vi "pco.camera_Live_Example_IMAQ - Copy.vi"() -> ()   [LabVIEW 2020]
doc: "A short program to demonstrate the fundamentals of control and image acquision with the pco.camera series. The program records a sequence of images, with \"live\" updating, until the \"StopRecording\" button is pressed. Use ctrl-H for more help on the individual controls and indicators.\n\nCopyright 2004, 2010 The Cooke Corporation."
uses:
  Camera.lvclass
  TimingControl.lvlib
panel:
  in  "Trigger":bool
  in  "data_format":T1(ring)=enum."Mono16"
  out "Image":T2(plugin-control)
  out "rawImage":u16[][](array[numeric])
  in  "Image Index":u32 max=9
  out "Recorded Images":u32
  in  "TriggerMode":T3(ring)
  in  "Quit":bool
  out "Error":errorcluster {"code" format="%x"}
  in  "Stop Record":bool
  out "Recording On":bool
  in  "roiY1":u64=2 min=1 max=1040 step=1
  in  "roiX1":u64=2 min=1 max=1392 step=1
  in  "roiY0":u64=1 min=1 max=1039 step=1
  in  "roiX0":u64=1 min=1 max=1391 step=1
  out "Image Height":u64
  out "Image Width":u64
  in  "dwImgCount":u32=10 caption="Required Number of Images" max=2397
  in  "Exposure Time [s]":dbl=0.010000000000000002 min=1e-06 max=60.0 step=0.001
  # "This example demonstrates the image acquisition with one camera in ring buffer mode together with a live display of the latest images during record. After record is stopped, the images can be addressed by index.\nNote that this example will not be fail save, i.e. doesnt react on errors, just handles them forward to the end\n\nUsage:\nSelect your required image count, data format and the camera setup before you start the program.\nOnce started, the camera class will be initialized and images will be recorded and displayed automatically\nYou can stop the images by pressing stop record.\nAfter stopped, the image at the selected index will be read out\nTo finish the program click on quit application, this will force an exit of the camera class\nYou can change your required ROI after and also during the record."
  # "pco.labview"
  # "Camera Setup"
  # "Recording Control"
  # "Parameters for image readout"
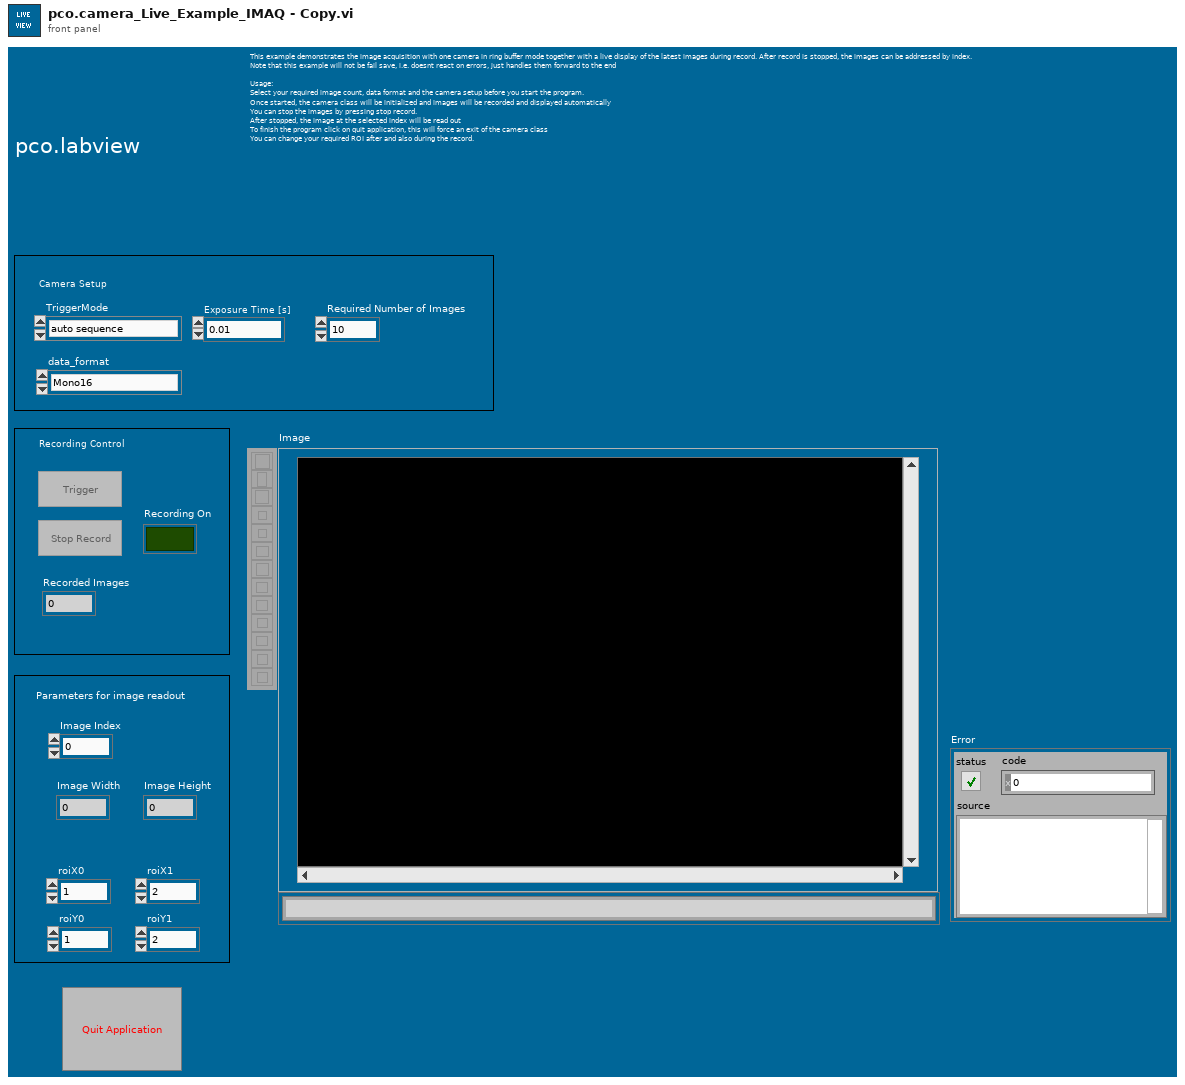
[diagram p1: front panel]
types:
  T1 = enum16{"Undefined", "Mono8", "Mono16", "BGRA8", "RGBA8", "BGRA16", "RGBA16", "CompressedMono8"}
  T2 = typedef "IMAQ Image.ctl" = refnum<image>
  T3 = enum16{"auto sequence", "software trigger", "external exposure start", "external exposure control"}
  T4 = enum16{"sequence", "sequence non blocking", "ring buffer", "fifo", "sequence_dpcore", "sequence_non_blocking_dpcore", "ring_buffer_dpcore", "fifo_dpcore", "tif", "multitif", "pcoraw", "b16", "dicom", "multidicom"}
  T5 = enum8{"Enabled", "Disabled", "Disabled and Grayed Out"}
  T6 = cluster{"serial":u32, "type":u16, "sub_type":u16, "interface_type":u16, "bit_resolution":u16, "min_exposure_time_s":dbl, "max_exposure_time_s":dbl, "min_exposure_step_s":dbl, "min_delay_time_s":dbl, "max_delay_time_s":dbl, "min_delay_step_s":dbl, "min_width":u64, "min_height":u64, "max_width":u64, "max_height":u64, "roi_step_horz":u64, "roi_step_vert":u64, "roi_symmetric_horz":bool, "roi_symmetric_vert":bool, "has_timestamp_mode":bool, "has_timestamp_mode_ascii_only":bool, "pixelrate_vec":u32[], "has_acquire_mode":bool, "has_ext_acquire_mode":bool, "has_metadata_mode":bool, "has_ram":bool, "binning_horz_vec":u16[], "binning_vert_vec":u16[]}
  T7 = typedef "Image Type" = u32
  T8 = typedef "Camera.lvclass/binning.ctl" = cluster{"vert":u16, "horz":u16}
  T9 = cluster{"exposure_time_s":dbl, "delay_time_s":dbl, "roi":cluster{"x0":u64, "y0":u64, "x1":u64, "y1":u64}, "timestamp_mode":u16, "pixelrate":u32, "trigger_mode":u16, "acquire_mode":u16, "metadata_mode":u16, "noisefilter_mode":u16, "binning":T8}
  T10 = cluster{"Plane 4 (alpha)":u16, "Plane 1 (Red)":u16, "Plane 2 (Green)":u16, "Plane 3 (Blue)":u16}[][]
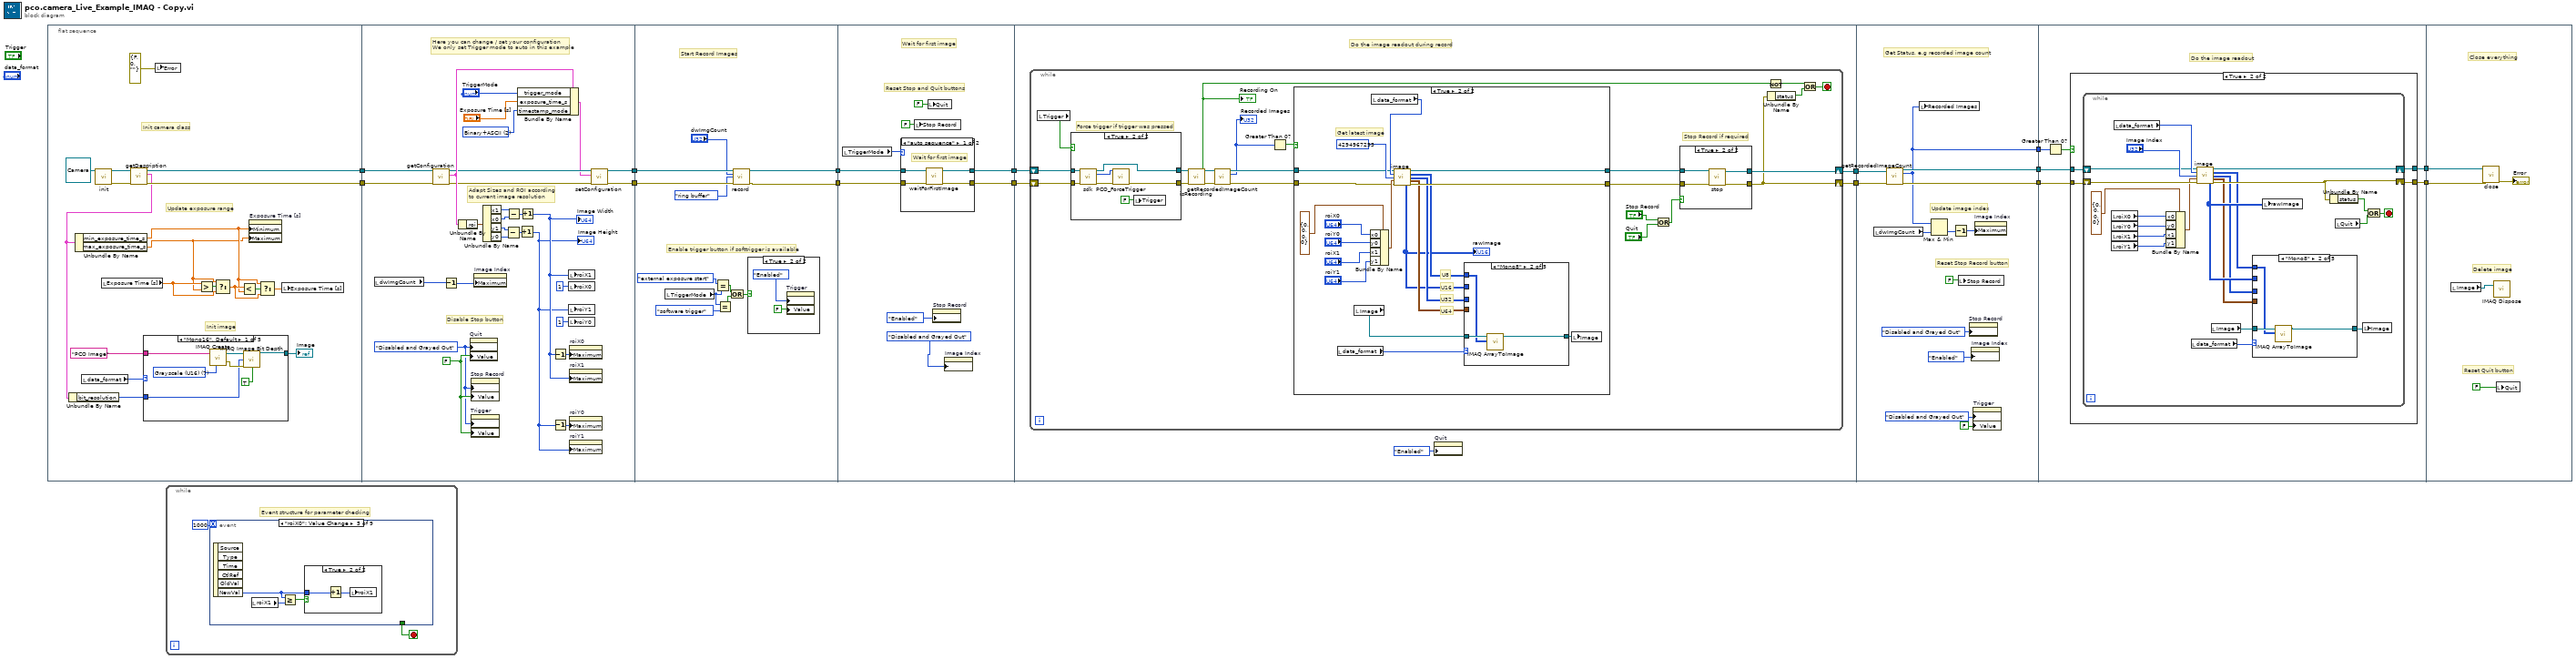
[diagram p0: block diagram]
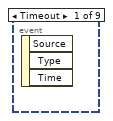
[diagram p2: hidden frame]
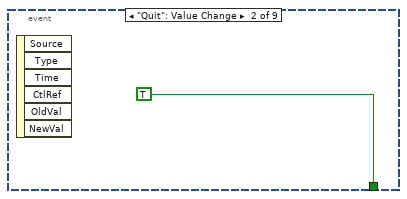
[diagram p3: hidden frame]
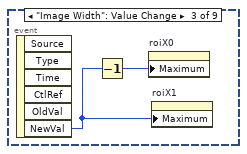
[diagram p4: hidden frame]
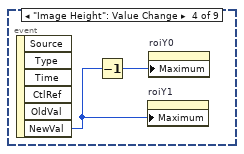
[diagram p5: hidden frame]
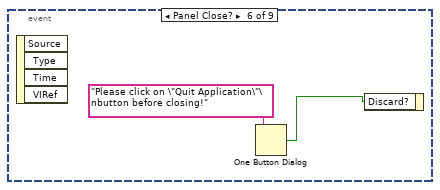
[diagram p7: hidden frame]
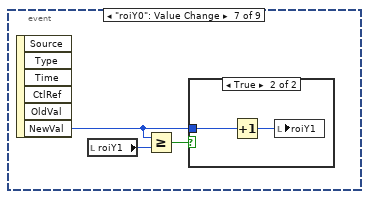
[diagram p8: hidden frame]
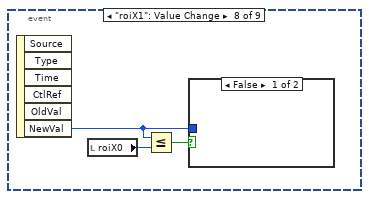
[diagram p10: hidden frame]
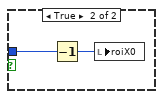
[diagram p11: hidden frame]
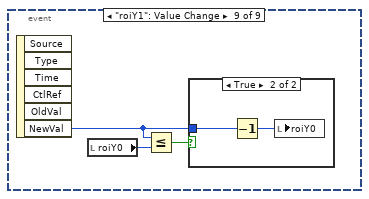
[diagram p12: hidden frame]
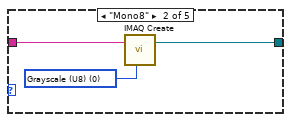
[diagram p14: hidden frame]
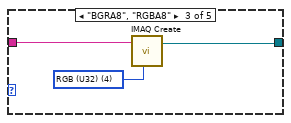
[diagram p15: hidden frame]
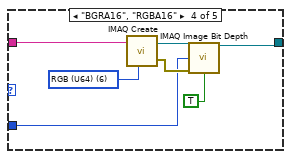
[diagram p16: hidden frame]
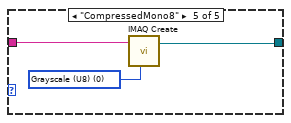
[diagram p17: hidden frame]
diagram:
  n1 = flat-sequence {
    tunnel: [w22] -> w7
    tunnel: [w21] -> w6
    tunnel: [w61] -> w15
    tunnel: [w65] -> w14
    tunnel: w7 -> [w60]
    tunnel: w6 -> [w59]
    tunnel: [w85] -> w9
    tunnel: [w86] -> w8
    tunnel: w14 -> [w96]
    tunnel: w15 -> [w95]
    tunnel: w9 -> [w103]
    tunnel: w8 -> [w104]
    tunnel: [w102] -> w13
    tunnel: [w100] -> w2
    tunnel: w13 -> [w118]
    tunnel: [w116] -> w12
    tunnel: [w115] -> w5
    tunnel: w2 -> [w114]
    tunnel: w12 -> [w201]
    tunnel: [w199] -> w11
    tunnel: w5 -> [w194]
    tunnel: [w193] -> w4
    tunnel: [w192] -> w1
    tunnel: w11 -> [w210]
    tunnel: [w209] -> w10
    tunnel: w4 -> [w208]
    tunnel: [w207] -> w3
    tunnel: w1 -> [w205]
    tunnel: w10 -> [w257]
    tunnel: w3 -> [w255]
    frame #0 {
      # "Init image"
      # "Init camera class"
      # "Update exposure range"
      n2 = local read "data_format"() -> (w18:T1)
      n3 = call-dynamic "init.vi"("Camera in"=refnum<class "Camera.lvclass"> refnum) -> ("Camera out"=w23:refnum<class "Camera.lvclass">, "error out"=w24:errorcluster)  [unwired: 8 in]
      n4 = local read "Exposure Time [s]"() -> (w32:dbl)
      n5 = call-dynamic "getDescription.vi"("error in (no error)"=w24, "Camera in"=w23) -> ("error out"=w21:errorcluster, "description"=w17:T6, "Camera out"=w22:refnum<class "Camera.lvclass">)  [unwired: 7 in]
      n6 = Unbundle By Name(w17) -> ("bit_resolution"=w16:u16)
      n7 = Unbundle By Name(w17) -> ("min_exposure_time_s"=w20:dbl, "max_exposure_time_s"=w19:dbl)
      n8 = case shown="\"Mono16\", Default" w18 {
        tunnel: "PCO Image" ("Image Name") -> [w39 w43 w45 w52 w55]
        tunnel: [w35 w41 w44 w49 w54] -> w25
        tunnel: w16 -> [w34 _ _ w47 _]
        frame "Mono16", Default {
          w40 = T7 7 items=["Grayscale (U8)", "Grayscale (I16)", "Grayscale (SGL)", "Complex (CSG)", "RGB (U32)", "HSL (U32)", "RGB (U64)", "Grayscale (U16)"] ("Image Type")
          n9 = call "IMAQ Create"("Image Name"=w39, "Image Type"=w40) -> ("New Image"=w37:T2, "error out"=w36:errorcluster)  [unwired: 3 in]
          n10 = call "IMAQ Image Bit Depth"("Image"=w37, "Bit Depth (0)"=w34, "error in (no error)"=w36, "Get/Set Bit Depth? (Set)"=TRUE) -> ("Image Out"=w35:T2)  [unwired: 9 in, 2 out]
        }
        frame "Mono8" {
          w42 = T7 0 items=["Grayscale (U8)", "Grayscale (I16)", "Grayscale (SGL)", "Complex (CSG)", "RGB (U32)", "HSL (U32)", "RGB (U64)", "Grayscale (U16)"] ("Image Type")
          n11 = call "IMAQ Create"("Image Name"=w43, "Image Type"=w42) -> ("New Image"=w41:T2)  [unwired: 3 in, 1 out]
        }
        frame "BGRA8", "RGBA8" {
          w46 = T7 4 items=["Grayscale (U8)", "Grayscale (I16)", "Grayscale (SGL)", "Complex (CSG)", "RGB (U32)", "HSL (U32)", "RGB (U64)", "Grayscale (U16)"] ("Image Type")
          n12 = call "IMAQ Create"("Image Name"=w45, "Image Type"=w46) -> ("New Image"=w44:T2)  [unwired: 3 in, 1 out]
        }
        frame "BGRA16", "RGBA16" {
          w53 = T7 6 items=["Grayscale (U8)", "Grayscale (I16)", "Grayscale (SGL)", "Complex (CSG)", "RGB (U32)", "HSL (U32)", "RGB (U64)", "Grayscale (U16)"] ("Image Type")
          n13 = call "IMAQ Create"("Image Name"=w52, "Image Type"=w53) -> ("New Image"=w50:T2, "error out"=w48:errorcluster)  [unwired: 3 in]
          n14 = call "IMAQ Image Bit Depth"("Image"=w50, "Bit Depth (0)"=w47, "error in (no error)"=w48, "Get/Set Bit Depth? (Set)"=TRUE) -> ("Image Out"=w49:T2)  [unwired: 9 in, 2 out]
        }
        frame "CompressedMono8" {
          w56 = T7 0 items=["Grayscale (U8)", "Grayscale (I16)", "Grayscale (SGL)", "Complex (CSG)", "RGB (U32)", "HSL (U32)", "RGB (U64)", "Grayscale (U16)"] ("Image Type")
          n15 = call "IMAQ Create"("Image Name"=w55, "Image Type"=w56) -> ("New Image"=w54:T2)  [unwired: 3 in, 1 out]
        }
      }
      "Image" <- w25
      n16 = local write "Error"(errorcluster {"status"=FALSE, "code"=0, "source"=""} ("error IO")) -> ()
      n17 = Greater?(x=w32, y=w19) -> (0:w33:bool)
      n18 = Select(t=w19, s=w33, f=w32) -> (s? t:f=w30:dbl)
      n19 = Less?(x=w30, y=w20) -> (x < y?=w31:bool)
      n20 = property on="Exposure Time [s]" class="DigNum (strict)"("Minimum"=w20, "Maximum"=w19) -> ()  [unwired: 2 in, 2 out]
      n21 = Select(t=w20, s=w31, f=w30) -> (s? t:f=w29:dbl)
      n22 = local write "Exposure Time [s]"(w29) -> ()
    }
    frame #1 {
      w71 = u16 2 items=["OFF", "Binary", "Binary+ASCII", "ASCII"] ("wTimeStampMode")
      w58 = FALSE ("Stop")
      w57 = T5."Disabled and Grayed Out" ("Disabled")
      # "Disable Stop button"
      # "Adapt Sizes and ROI according\nto current image resolution"
      # "Here you can change / set your configuration\nWe only set Trigger mode to auto in this example"
      n23 = local read "dwImgCount"() -> (w72:u32)
      n24 = call-dynamic "getConfiguration.vi"("error in (no error)"=w59, "Camera in"=w60) -> ("error out"=w66:errorcluster, "configuration"=w77:T9, "Camera out"=w68:refnum<class "Camera.lvclass">)  [unwired: 7 in]
      n25 = Decrement(x=w72) -> (x-1=w62:u32)
      n26 = Unbundle By Name(w77) -> ("roi"=w78:cluster{"x0":u64, "y0":u64, "x1":u64, "y1":u64})
      n27 = property on="Quit" class="Bool (strict)"("DisabledEnum"=w57, "Value"=w58) -> ()  [unwired: 2 in, 2 out]
      n28 = property on="Stop Record" class="Bool (strict)"("DisabledEnum"=w57, "Value"=w58) -> ()  [unwired: 2 in, 2 out]
      n29 = property on="Trigger" class="Bool (strict)"("DisabledEnum"=w57, "Value"=w58) -> ()  [unwired: 2 in, 2 out]
      n30 = property on="Image Index" class="DigNum (strict)"("Maximum"=w62) -> ()  [unwired: 2 in, 2 out]
      n31 = Unbundle By Name(w78) -> ("x1"=w80:u64, "x0"=w79:u64, "y1"=w82:u64, "y0"=w81:u64)
      n32 = Subtract(x=w82, y=w81) -> (x-y=w84:u64)
      n33 = Subtract(x=w80, y=w79) -> (x-y=w83:u64)
      n34 = Bundle By Name(cluster=w77, "trigger_mode"="TriggerMode", "exposure_time_s"="Exposure Time [s]", "timestamp_mode"=w71) -> (w67:T9)
      n35 = Increment(x=w84) -> (x+1=w63:u64)
      "Image Height" <- w63
      n36 = Increment(x=w83) -> (x+1=w64:u64)
      "Image Width" <- w64
      n37 = Decrement(x=w64) -> (x-1=w75:u64)
      n38 = Decrement(x=w63) -> (x-1=w76:u64)
      n39 = local write "roiX1"(w64) -> ()
      n40 = local write "roiX0"(u64 1 ("roiY0")) -> ()
      n41 = local write "roiY1"(w63) -> ()
      n42 = local write "roiY0"(u64 1 ("roiY0")) -> ()
      n43 = property on="roiX0" class="DigNum (strict)"("Maximum"=w75) -> ()  [unwired: 2 in, 2 out]
      n44 = property on="roiX1" class="DigNum (strict)"("Maximum"=w64) -> ()  [unwired: 2 in, 2 out]
      n45 = property on="roiY0" class="DigNum (strict)"("Maximum"=w76) -> ()  [unwired: 2 in, 2 out]
      n46 = property on="roiY1" class="DigNum (strict)"("Maximum"=w63) -> ()  [unwired: 2 in, 2 out]
      n47 = call-dynamic "setConfiguration.vi"("error in (no error)"=w66, "configuration"=w67, "Camera in"=w68) -> ("error out"=w65:errorcluster, "Camera out"=w61:refnum<class "Camera.lvclass">)  [unwired: 7 in]
    }
    frame #2 {
      # "Enable trigger button if softtrigger is available"
      # "Start Record Images"
      n48 = local read "TriggerMode"() -> (w92:T3)
      n49 = Equal?(x=T3."external exposure start" ("TriggerMode"), y=w92) -> (x = y?=w89:bool)
      n50 = Equal?(x=w92, y=T3."software trigger" ("TriggerMode")) -> (x = y?=w88:bool)
      n51 = Or(x=w89, y=w88) -> (x .or. y?=w90:bool)
      n52 = call-dynamic "record.vi"("Camera in"=w95, "num_images"="dwImgCount", "record_mode"=T4."ring buffer", "error in (no error)"=w96) -> ("Camera out"=w86:refnum<class "Camera.lvclass">, "error out"=w85:errorcluster)  [unwired: 10 in]
      n53 = case shown="True" w90 {
        frame False {
        }
        frame True {
          n54 = property on="Trigger" class="Bool (strict)"("DisabledEnum"=T5."Enabled" ("Disabled"), "Value"=FALSE ("Trigger")) -> ()  [unwired: 2 in, 2 out]
        }
      }
    }
    frame #3 {
      # "Wait for first image"
      # "Reset Stop and Quit buttons"
      n55 = local read "TriggerMode"() -> (w99:T3)
      n56 = case shown="\"auto sequence\"" w99 {
        tunnel: w104 -> [w111 w113]
        tunnel: w103 -> [w110 w112]
        tunnel: [w109 w112] -> w102
        tunnel: [w108 w113] -> w100
        frame "auto sequence" {
          # "Wait for first image"
          n57 = call-dynamic "waitForFirstImage.vi"("error in (no error)"=w110, "Camera in"=w111) -> ("error out"=w109:errorcluster, "Camera out"=w108:refnum<class "Camera.lvclass">)  [unwired: 8 in]
        }
        frame Default {
        }
      }
      n58 = local write "Stop Record"(FALSE ("Stop Record")) -> ()
      n59 = local write "Quit"(FALSE ("Stop")) -> ()
      n60 = property on="Stop Record" class="Bool (strict)"("DisabledEnum"=T5."Enabled" ("Disabled")) -> ()  [unwired: 2 in, 2 out]
      n61 = property on="Image Index" class="DigNum (strict)"("DisabledEnum"=T5."Disabled and Grayed Out" ("Disabled")) -> ()  [unwired: 2 in, 2 out]
    }
    frame #4 {
      # "Do the image readout during record"
      n62 = while {
        shift-right: [w121] -> w116
        shift-left: w118 -> [w125]
        shift-right: [w122] -> w115
        shift-left: w114 -> [w126]
        stop <- w137 stop-if-true
        # "Force trigger if trigger was pressed"
        # "Stop Record if required"
        n63 = local read "Trigger"() -> (w127:bool)
        n64 = case shown="True" w127 {
          tunnel: w126 -> [w178 w183]
          tunnel: w125 -> [w177 w182]
          tunnel: [w178 w181] -> w124
          tunnel: [w177 w180] -> w123
          frame False {
          }
          frame True {
            n65 = call-dynamic "sdk.vi"("Camera in"=w183, "error in (no error)"=w182) -> ("Camera out"=w181:refnum<class "Camera.lvclass">, "sdk"=w184:u64, "error out"=w185:errorcluster)  [unwired: 11 in]
            n66 = call "PCO_ForceTrigger.vi"("error in (no error)"=w185, "ph"=w184) -> ("error out"=w180:errorcluster)  [unwired: 6 in, 3 out]
            n67 = local write "Trigger"(FALSE ("Trigger")) -> ()
          }
        }
        n68 = call-dynamic "isRecording.vi"("Camera in"=w124, "error in (no error)"=w123) -> ("Camera out"=w132:refnum<class "Camera.lvclass">, "recording"=w135:bool, "error out"=w131:errorcluster)  [unwired: 11 in]
        "Recording On" <- w135
        n69 = call-dynamic "getRecordedImageCount.vi"("Camera in"=w132, "error in (no error)"=w131) -> ("Camera out"=w129:refnum<class "Camera.lvclass">, "recorded_image_count"=w119:u32, "error out"=w130:errorcluster)  [unwired: 11 in]
        "Recorded Images" <- w119
        n70 = Greater Than 0?(x=w119) -> (x > 0?=w120:bool)
        n71 = case shown="True" w120 {
          tunnel: [w141 w156] -> w133
          tunnel: w130 -> [w141 w153]
          tunnel: w129 -> [w142 w144]
          tunnel: [w142 w143] -> w128
          frame False {
          }
          frame True {
            # "U64"
            # "U32"
            # "U8"
            # "U16"
            # "Get latest image"
            n72 = local read "data_format"() -> (w145:T1)
            n73 = local read "Image"() -> (w150:T2)
            n74 = Bundle By Name(cluster=cluster{"x0":u64, "y0":u64, "x1":u64, "y1":u64} {"x0"=0, "y0"=0, "x1"=0, "y1"=0} ("roi"), "x0"="roiX0", "y0"="roiY0", "x1"="roiX1", "y1"="roiY1") -> (w157:cluster{"x0":u64, "y0":u64, "x1":u64, "y1":u64})
            n75 = local read "data_format"() -> (w152:T1)
            n76 = call-dynamic "image.vi"("Camera in"=w144, "data_format"=w152, "image_index"=u32 4294967295 ("dwImgIdx"), "roi"=w157, "error in (no error)"=w153) -> ("Camera out"=w143:refnum<class "Camera.lvclass">, "image (U8)"=w147:u8[][], "image (U32)"=w148:u32[][], "image (U64)"=w149:T10, "raw_image (U16)"=w146:u16[][], "error out"=w156:errorcluster)  [unwired: 3 in, 2 out]
            "rawImage" <- w146
            n77 = case shown="\"Mono8\"" w145 {
              tunnel: w150 -> [w164 w167 w170 w173 w176]
              tunnel: [w162 w165 w169 w171 w175] -> w151
              tunnel: w149 -> [_ _ _ w172 _]
              tunnel: w148 -> [_ _ w168 _ _]
              tunnel: w147 -> [_ w166 _ _ w174]
              tunnel: w146 -> [w163 _ _ _ _]
              frame "Mono16", Default {
                n78 = call "IMAQ ArrayToImage"("Image Pixels (U16)"=w163, "Image"=w164) -> ("Image Out"=w162:T2)  [unwired: 8 in, 1 out]
              }
              frame "Mono8" {
                n79 = call "IMAQ ArrayToImage"("Image Pixels (U8)"=w166, "Image"=w167) -> ("Image Out"=w165:T2)  [unwired: 8 in, 1 out]
              }
              frame "BGRA8", "RGBA8" {
                n80 = call "IMAQ ArrayToColorImage"("Image Pixels (U32)"=w168, "Image"=w170) -> ("Image Out"=w169:T2)  [unwired: 3 in, 1 out]
              }
              frame "BGRA16", "RGBA16" {
                n81 = call "IMAQ ArrayToColorImage"("Image"=w173, "Image Pixels (U64)"=w172) -> ("Image Out"=w171:T2)  [unwired: 3 in, 1 out]
              }
              frame "CompressedMono8" {
                n82 = call "IMAQ ArrayToImage"("Image Pixels (U8)"=w174, "Image"=w176) -> ("Image Out"=w175:T2)  [unwired: 8 in, 1 out]
              }
            }
            n83 = local write "Image"(w151) -> ()
          }
        }
        n84 = Or(x="Stop Record", y="Quit") -> (x .or. y?=w138:bool)
        n85 = case shown="True" w138 {
          tunnel: w133 -> [w187 w188]
          tunnel: [w186 w190] -> w122
          tunnel: [w187 w191] -> w121
          tunnel: w128 -> [w186 w189]
          frame False {
          }
          frame True {
            n86 = call-dynamic "stop.vi"("error in (no error)"=w188, "Camera in"=w189) -> ("error out"=w191:errorcluster, "Camera out"=w190:refnum<class "Camera.lvclass">)  [unwired: 8 in]
          }
        }
        n87 = Unbundle By Name(w121) -> ("status"=w136:bool)
        n88 = Not(x=w135) -> (.not. x?=w134:bool)
        n89 = Or(x=w134, y=w136) -> (x .or. y?=w137:bool)
      }
      n90 = property on="Quit" class="Bool (strict)"("DisabledEnum"=T5."Enabled" ("Disabled")) -> ()  [unwired: 2 in, 2 out]
    }
    frame #5 {
      # "Update image index"
      # "Reset Stop Record button"
      # "Get Status, e.g recorded image count"
      n91 = local read "dwImgCount"() -> (w200:u32)
      n92 = call-dynamic "getRecordedImageCount.vi"("Camera in"=w194, "error in (no error)"=w201) -> ("Camera out"=w193:refnum<class "Camera.lvclass">, "recorded_image_count"=w192:u32, "error out"=w199:errorcluster)  [unwired: 11 in]
      n93 = local write "Recorded Images"(w192) -> ()
      n94 = Max & Min(x=w192, y=w200) -> (min(x,y)=w202:u32)  [unwired: 1 out]
      n95 = Decrement(x=w202) -> (x-1=w197:u32)
      n96 = local write "Stop Record"(FALSE ("Stop Record")) -> ()
      n97 = property on="Stop Record" class="Bool (strict)"("DisabledEnum"=T5."Disabled and Grayed Out" ("Disabled")) -> ()  [unwired: 2 in, 2 out]
      n98 = property on="Image Index" class="DigNum (strict)"("DisabledEnum"=T5."Enabled" ("Disabled")) -> ()  [unwired: 2 in, 2 out]
      n99 = property on="Trigger" class="Bool (strict)"("DisabledEnum"=T5."Disabled and Grayed Out" ("Disabled"), "Value"=FALSE ("Trigger")) -> ()  [unwired: 2 in, 2 out]
      n100 = property on="Image Index" class="DigNum (strict)"("Maximum"=w197) -> ()  [unwired: 2 in, 2 out]
    }
    frame #6 {
      # "Do the image readout"
      n101 = Greater Than 0?(x=w205) -> (x > 0?=w206:bool)
      n102 = case shown="True" w206 {
        tunnel: w210 -> [w211 w216]
        tunnel: [w211 w215] -> w209
        tunnel: w208 -> [w212 w214]
        tunnel: [w212 w213] -> w207
        frame False {
        }
        frame True {
          n103 = while {
            shift-right: [w230] -> w215
            shift-left: w216 -> [w238]
            shift-right: [w217] -> w213
            shift-left: w214 -> [w218]
            stop <- w232 stop-if-true
            n104 = local read "roiX0"() -> (w228:u64)
            n105 = local read "roiY0"() -> (w229:u64)
            n106 = local read "roiX1"() -> (w236:u64)
            n107 = local read "roiY1"() -> (w235:u64)
            n108 = local read "data_format"() -> (w226:T1)
            n109 = Bundle By Name(cluster=cluster{"x0":u64, "y0":u64, "x1":u64, "y1":u64} {"x0"=0, "y0"=0, "x1"=0, "y1"=0} ("roi"), "x0"=w228, "y0"=w229, "x1"=w236, "y1"=w235) -> (w237:cluster{"x0":u64, "y0":u64, "x1":u64, "y1":u64})
            n110 = local read "data_format"() -> (w219:T1)
            n111 = call-dynamic "image.vi"("Camera in"=w218, "data_format"=w226, "image_index"="Image Index", "roi"=w237, "error in (no error)"=w238) -> ("Camera out"=w217:refnum<class "Camera.lvclass">, "image (U8)"=w222:u8[][], "image (U32)"=w221:u32[][], "image (U64)"=w220:T10, "raw_image (U16)"=w223:u16[][], "error out"=w230:errorcluster)  [unwired: 3 in, 2 out]
            n112 = local read "Image"() -> (w224:T2)
            n113 = case shown="\"Mono8\"" w219 {
              tunnel: w224 -> [w241 w244 w247 w250 w253]
              tunnel: [w239 w242 w246 w248 w252] -> w225
              tunnel: w220 -> [_ _ _ w249 _]
              tunnel: w221 -> [_ _ w245 _ _]
              tunnel: w222 -> [_ w243 _ _ w251]
              tunnel: w223 -> [w240 _ _ _ _]
              frame "Mono16", Default {
                n114 = call "IMAQ ArrayToImage"("Image Pixels (U16)"=w240, "Image"=w241) -> ("Image Out"=w239:T2)  [unwired: 8 in, 1 out]
              }
              frame "Mono8" {
                n115 = call "IMAQ ArrayToImage"("Image Pixels (U8)"=w243, "Image"=w244) -> ("Image Out"=w242:T2)  [unwired: 8 in, 1 out]
              }
              frame "BGRA8", "RGBA8" {
                n116 = call "IMAQ ArrayToColorImage"("Image Pixels (U32)"=w245, "Image"=w247) -> ("Image Out"=w246:T2)  [unwired: 3 in, 1 out]
              }
              frame "BGRA16", "RGBA16" {
                n117 = call "IMAQ ArrayToColorImage"("Image"=w250, "Image Pixels (U64)"=w249) -> ("Image Out"=w248:T2)  [unwired: 3 in, 1 out]
              }
              frame "CompressedMono8" {
                n118 = call "IMAQ ArrayToImage"("Image Pixels (U8)"=w251, "Image"=w253) -> ("Image Out"=w252:T2)  [unwired: 8 in, 1 out]
              }
            }
            n119 = local write "rawImage"(w223) -> ()
            n120 = Unbundle By Name(w230) -> ("status"=w233:bool)
            n121 = local read "Quit"() -> (w234:bool)
            n122 = local write "Image"(w225) -> ()
            n123 = Or(x=w233, y=w234) -> (x .or. y?=w232:bool)
          }
        }
      }
    }
    frame #7 {
      # "Delete image"
      # "Close everything"
      # "Reset Quit button"
      n124 = local read "Image"() -> (w254:T2)
      n125 = call-dynamic "close.vi"("error in (no error)"=w257, "Camera in"=w255) -> ("error out"=→"Error":errorcluster)  [unwired: 9 in]
      n126 = call "IMAQ Dispose"("Image"=w254) -> ()  [unwired: 5 in, 1 out]
      n127 = local write "Quit"(FALSE ("Stop Record")) -> ()
    }
  }
  n128 = while {
    stop <- w259 stop-if-true
    # "Event structure for parameter checking"
    n129 = event shown="[4] \"roiX0\": Value Change" {
      selector: _ -> [_ _ _ _ _ _ _ _ _]
      dyn-events: _ -> [_ _ _ _ _ _ _ _ _]
      timeout: 1000 -> [_ _ _ _ _ _ _ _ _]
      tunnel: [_ TRUE _ _ _ _ _ _ _] -> w259
      event Timeout {
        n130 = event-data() -> ()  [unwired: 1 in, 3 out]
      }
      event "Quit": Value Change {
        n131 = event-data() -> ()  [unwired: 1 in, 6 out]
      }
      event "Image Width": Value Change {
        n132 = event-data() -> ("NewVal"=w262:u64)  [unwired: 1 in, 5 out]
        n133 = Decrement(x=w262) -> (x-1=w263:u64)
        n134 = property on="roiX0" class="DigNum (strict)"("Maximum"=w263) -> ()  [unwired: 2 in, 2 out]
        n135 = property on="roiX1" class="DigNum (strict)"("Maximum"=w262) -> ()  [unwired: 2 in, 2 out]
      }
      event "Image Height": Value Change {
        n136 = event-data() -> ("NewVal"=w264:u64)  [unwired: 1 in, 5 out]
        n137 = Decrement(x=w264) -> (x-1=w265:u64)
        n138 = property on="roiY1" class="DigNum (strict)"("Maximum"=w264) -> ()  [unwired: 2 in, 2 out]
        n139 = property on="roiY0" class="DigNum (strict)"("Maximum"=w265) -> ()  [unwired: 2 in, 2 out]
      }
      event "roiX0": Value Change {
        n140 = event-data() -> ("NewVal"=w266:u64)  [unwired: 1 in, 5 out]
        n141 = local read "roiX1"() -> (w268:u64)
        n142 = Greater Or Equal?(x=w266, y=w268) -> (x >= y?=w267:bool)
        n143 = case shown="True" w267 {
          tunnel: w266 -> [_ w270]
          frame False {
          }
          frame True {
            n144 = Increment(x=w270) -> (x+1=w269:u64)
            n145 = local write "roiX1"(w269) -> ()
          }
        }
      }
      event Panel Close? {
        n146 = event-data() -> ()  [unwired: 1 in, 4 out]
        n147 = One Button Dialog(message="Please click on \"Quit Application\"\nbutton before closing!") -> (true=w271:bool)  [unwired: 1 in]
        n148 = event-data("Discard?"=w271) -> ()  [unwired: 1 in, 1 out]
      }
      event "roiY0": Value Change {
        n149 = event-data() -> ("NewVal"=w273:u64)  [unwired: 1 in, 5 out]
        n150 = local read "roiY1"() -> (w275:u64)
        n151 = Greater Or Equal?(x=w273, y=w275) -> (x >= y?=w274:bool)
        n152 = case shown="True" w274 {
          tunnel: w273 -> [_ w277]
          frame False {
          }
          frame True {
            n153 = Increment(x=w277) -> (x+1=w276:u64)
            n154 = local write "roiY1"(w276) -> ()
          }
        }
      }
      event "roiX1": Value Change {
        n155 = event-data() -> ("NewVal"=w278:u64)  [unwired: 1 in, 5 out]
        n156 = local read "roiX0"() -> (w280:u64)
        n157 = Less Or Equal?(x=w278, y=w280) -> (x <= y?=w279:bool)
        n158 = case shown="False" w279 {
          tunnel: w278 -> [_ w282]
          frame False {
          }
          frame True {
            n159 = Decrement(x=w282) -> (x-1=w281:u64)
            n160 = local write "roiX0"(w281) -> ()
          }
        }
      }
      event "roiY1": Value Change {
        n161 = event-data() -> ("NewVal"=w283:u64)  [unwired: 1 in, 5 out]
        n162 = local read "roiY0"() -> (w285:u64)
        n163 = Less Or Equal?(x=w283, y=w285) -> (x <= y?=w284:bool)
        n164 = case shown="True" w284 {
          tunnel: w283 -> [_ w287]
          frame False {
          }
          frame True {
            n165 = Decrement(x=w287) -> (x-1=w286:u64)
            n166 = local write "roiY0"(w286) -> ()
          }
        }
      }
    }
  }
